vi "Generic Load.vi"() -> ()   [LabVIEW 2014]
panel:
  out "error out":errorcluster {"code" format="%.0x"}
  in  "resource name":refnum<k15>="GPIB::5::INSTR"
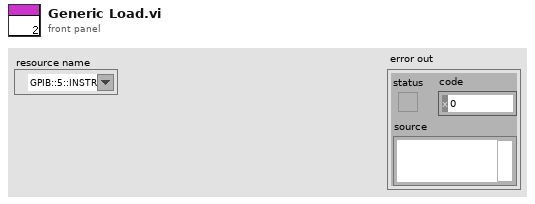
[diagram p1: front panel]
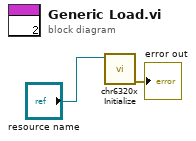
[diagram p0: block diagram]
diagram:
  n1 = call <instrlib>:"chr6320x Initialize.vi"("resource name"="resource name") -> ("error out"=→"error out":errorcluster)  [unwired: 9 in, 1 out]
